vi "Send to Database.vi"(7 "Setting Database In":refnum<class "Setting Database.lvclass">, 8 "error in":errorcluster, 11 "Archivist in":refnum<class "Archivist.lvclass">) -> (0 "error out":errorcluster, 3 "Archivist out":refnum<class "Archivist.lvclass">, 5 "Setting Database Out":refnum<class "Setting Database.lvclass">)   [LabVIEW 2019, in "Archivist.lvclass"]
uses:
  Archivist.lvclass
  Settings/Setting Database/Setting Database.lvclass
  Settings/Setting Database/Typedefs/PrivateEvents--Setting Database.Refresh.ctl
  Archivist.lvclass/Archivist.ctl
  Settings/Dot Settings/Dot Settings.lvclass
  C:/Users/Albro/Documents/GitHub/AFM-Lithography/lvsrc/Classes/Settings/ObjectSettings/ObjectSettings.lvclass
  Settings/Funnel Settings/Funnel Settings.lvclass
  Settings/Rectangle Settings/Rectangle Settings.lvclass
  Settings/Path Settings/Path Settings.lvclass
panel:
  out "Numeric 5":i32
  out "Numeric 4":i32
  out "Numeric 3":i32
  out "Numeric 2":i32
  out "Numeric":i32
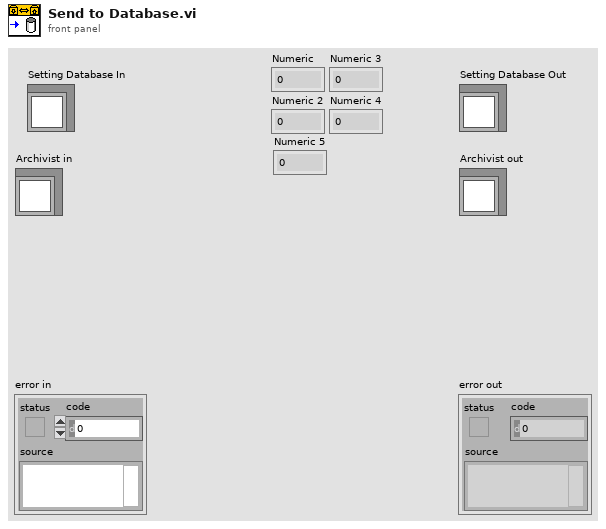
[diagram p1: front panel]
types:
  T1 = typedef "Setting Database.lvclass/PrivateEvents--Setting Database.Refresh.ctl" = cluster{"Paths":string[], "Rectangles":string[], "Funnels":string[], "Dots":string[]}
  T2 = typedef "Setting Database.lvclass/PublicEvents--Setting Database.PathsUpdated.ctl" = refnum<class "Path Settings.lvclass">[]
  T3 = typedef "Setting Database.lvclass/PublicEvents--Setting Database.RectanglesUpdated.ctl" = refnum<class "Rectangle Settings.lvclass">[]
  T4 = typedef "Setting Database.lvclass/PublicEvents--Setting Database.FunnelsUpdated.ctl" = refnum<class "Funnel Settings.lvclass">[]
  T5 = typedef "Setting Database.lvclass/PublicEvents--Setting Database.DotsUpdated.ctl" = refnum<class "Dot Settings.lvclass">[]
  T6 = typedef "Setting Database.lvclass/PublicEvents--Cluster.ctl" = cluster{"NewActivePath":refnum<user-event>, "PathsUpdated":refnum<user-event>, "RectanglesUpdated":refnum<user-event>, "NewActiveRectangle":refnum<user-event>, "NewActiveFunnel":refnum<user-event>, "FunnelsUpdated":refnum<user-event>, "NewActiveDot":refnum<user-event>, "DotsUpdated":refnum<user-event>}
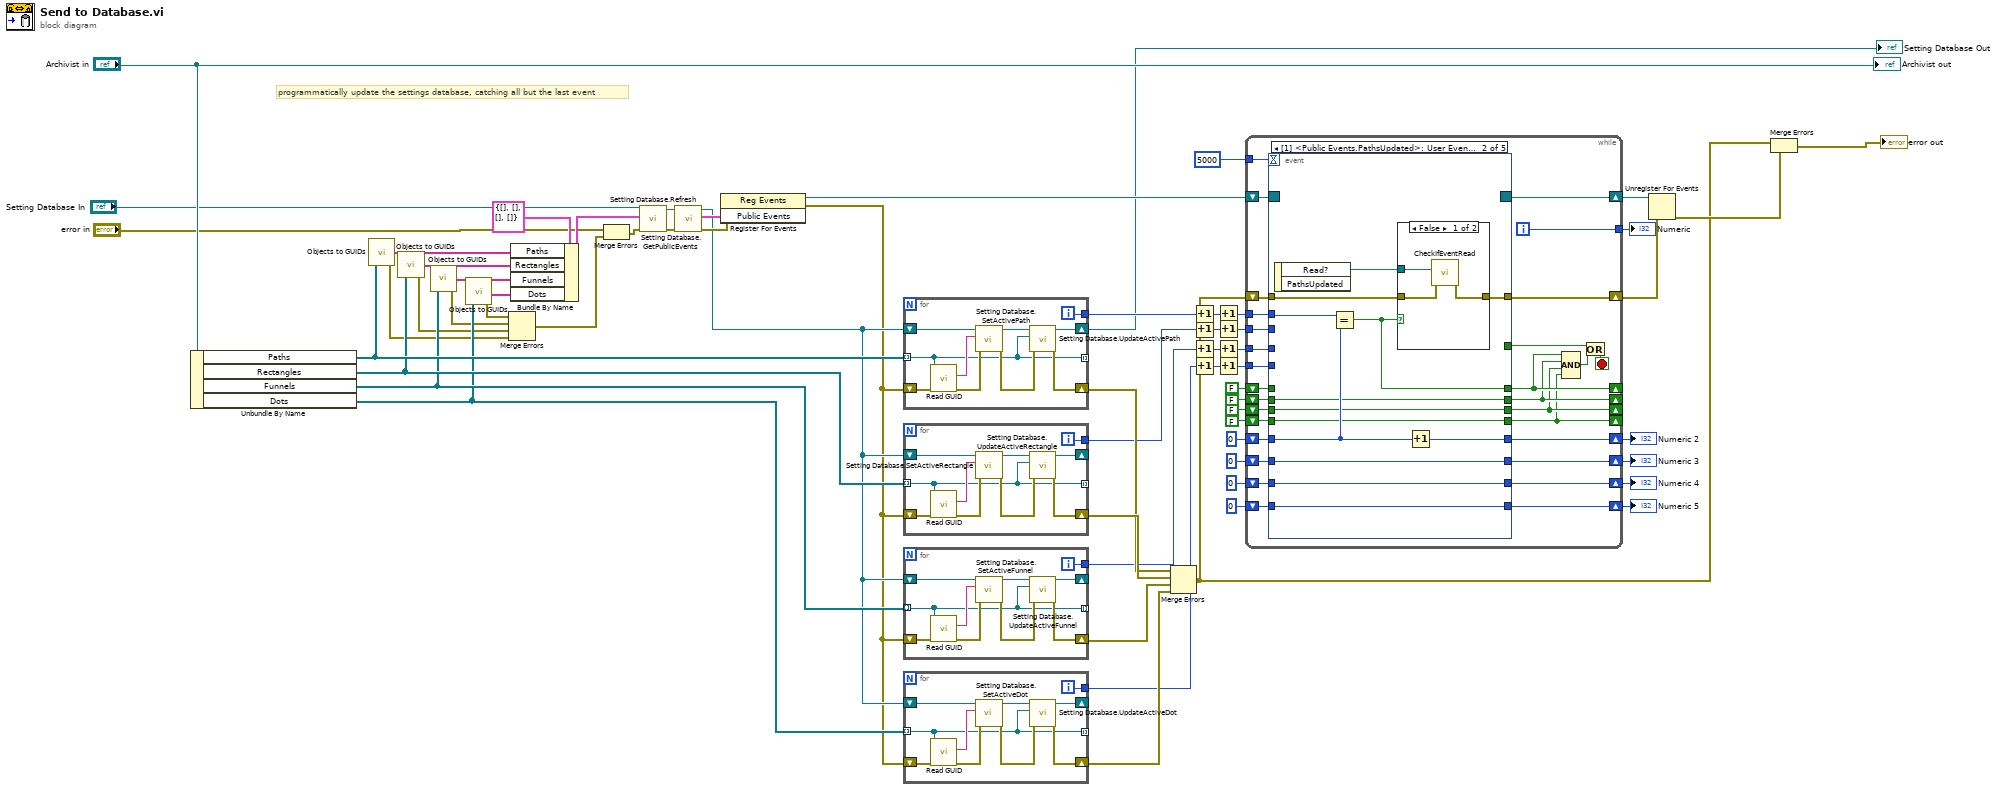
[diagram p0: block diagram]
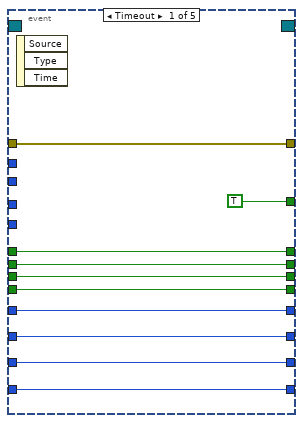
[diagram p2: hidden frame]
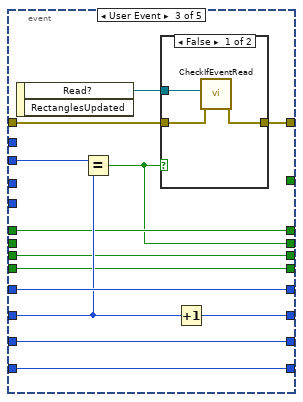
[diagram p4: hidden frame]
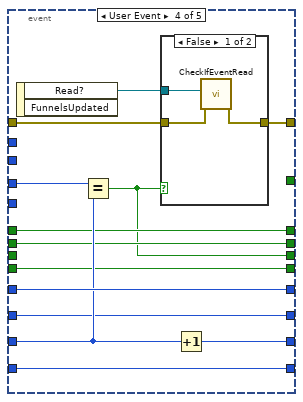
[diagram p6: hidden frame]
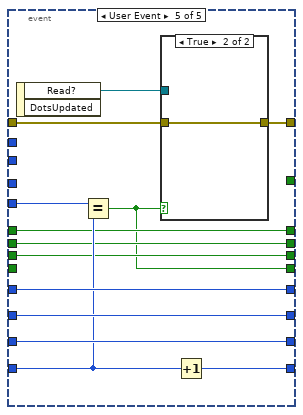
[diagram p8: hidden frame]
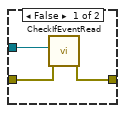
[diagram p9: hidden frame]
diagram:
  # "programmatically update the settings database, catching all but the last event"
  n1 = Unbundle By Name("Archivist in") -> ("Paths"=w51:T2, "Rectangles"=w43:T3, "Funnels"=w42:T4, "Dots"=w41:T5)
  n2 = call "Objects to GUIDs.vi"("Objects"=w51) -> ("error out"=w27:errorcluster, "GUIDs"=w59:string[])  [unwired: 3 in]
  n3 = call "Objects to GUIDs.vi"("Objects"=w43) -> ("error out"=w28:errorcluster, "GUIDs"=w50:string[])  [unwired: 3 in]
  n4 = call "Objects to GUIDs.vi"("Objects"=w42) -> ("error out"=w29:errorcluster, "GUIDs"=w49:string[])  [unwired: 3 in]
  n5 = call "Objects to GUIDs.vi"("Objects"=w41) -> ("error out"=w30:errorcluster, "GUIDs"=w48:string[])  [unwired: 3 in]
  n6 = Merge Errors(w30, w29, w28, w27) -> (w25:errorcluster)
  n7 = Bundle By Name(cluster=T1 {"Paths"=[], "Rectangles"=[], "Funnels"=[], "Dots"=[]} ("Initialize"), "Paths"=w59, "Rectangles"=w50, "Funnels"=w49, "Dots"=w48) -> (w58:T1)
  n8 = Merge Errors("error in", w25) -> (w26:errorcluster)
  n9 = call "Setting Database.Refresh.vi"("error in (no error)"=w26, "Initialize"=w58, "Setting Database"="Setting Database In") -> ("error out"=w45:errorcluster, "Setting Database out"=w46:refnum<class "Setting Database.lvclass">)  [unwired: 7 in]
  n10 = call "Setting Database.GetPublicEvents.vi"("error in (no error)"=w45, "Setting Database"=w46) -> ("error out"=w44:errorcluster, "Public Events"=w47:T6, "Setting Database out"=w40:refnum<class "Setting Database.lvclass">)  [unwired: 7 in]
  n11 = register-events(error in=w44, w47) -> (reference out=w62:refnum<event-registration>, error out=w39:errorcluster)  [unwired: 1 in]
  n12 = for {
    shift-right: [w71] -> w31
    shift-left: w40 -> [w70]
    shift-right: [w66] -> w52
    shift-left: w39 -> [w72]
    tunnel: w51 -> [w64] mode=indexing
    tunnel: [w64] -> _ mode=indexing
    tunnel: [w63] -> w57
    i -> [w63]
    n13 = call-dynamic "Read GUID.vi"("error in (no error)"=w72, "ObjectSettings in"=w64) -> ("error out"=w67:errorcluster, "GUID"=w65:string)  [unwired: 7 in, 1 out]
    n14 = call "Setting Database.SetActivePath.vi"("error in (no error)"=w67, "SetActivePath"=w65, "Setting Database"=w70) -> ("error out"=w68:errorcluster, "Setting Database out"=w69:refnum<class "Setting Database.lvclass">)  [unwired: 7 in]
    n15 = call "Setting Database.UpdateActivePath.vi"("error in (no error)"=w68, "UpdateCurrentPath"=w64, "Setting Database"=w69) -> ("error out"=w66:errorcluster, "Setting Database out"=w71:refnum<class "Setting Database.lvclass">)  [unwired: 7 in]
  }
  "Setting Database Out" <- w31
  n16 = for {
    shift-right: [w81] -> _
    shift-left: w40 -> [w80]
    shift-right: [w76] -> w55
    shift-left: w39 -> [w82]
    tunnel: w43 -> [w74] mode=indexing
    tunnel: [w74] -> _ mode=indexing
    tunnel: [w73] -> w38
    i -> [w73]
    n17 = call-dynamic "Read GUID.vi"("error in (no error)"=w82, "ObjectSettings in"=w74) -> ("error out"=w77:errorcluster, "GUID"=w75:string)  [unwired: 7 in, 1 out]
    n18 = call "Setting Database.SetActiveRectangle.vi"("error in (no error)"=w77, "SetActiveRectangle"=w75, "Setting Database"=w80) -> ("error out"=w78:errorcluster, "Setting Database out"=w79:refnum<class "Setting Database.lvclass">)  [unwired: 7 in]
    n19 = call "Setting Database.UpdateActiveRectangle.vi"("error in (no error)"=w78, "UpdateActiveRectangle"=w74, "Setting Database"=w79) -> ("error out"=w76:errorcluster, "Setting Database out"=w81:refnum<class "Setting Database.lvclass">)  [unwired: 7 in]
  }
  n20 = for {
    shift-right: [w91] -> _
    shift-left: w40 -> [w90]
    shift-right: [w86] -> w54
    shift-left: w39 -> [w92]
    tunnel: w42 -> [w84] mode=indexing
    tunnel: [w84] -> _ mode=indexing
    tunnel: [w83] -> w34
    i -> [w83]
    n21 = call-dynamic "Read GUID.vi"("error in (no error)"=w92, "ObjectSettings in"=w84) -> ("error out"=w87:errorcluster, "GUID"=w85:string)  [unwired: 7 in, 1 out]
    n22 = call "Setting Database.SetActiveFunnel.vi"("error in (no error)"=w87, "SetActiveFunnel"=w85, "Setting Database"=w90) -> ("error out"=w88:errorcluster, "Setting Database out"=w89:refnum<class "Setting Database.lvclass">)  [unwired: 7 in]
    n23 = call "Setting Database.UpdateActiveFunnel.vi"("error in (no error)"=w88, "UpdateActiveFunnel"=w84, "Setting Database"=w89) -> ("error out"=w86:errorcluster, "Setting Database out"=w91:refnum<class "Setting Database.lvclass">)  [unwired: 7 in]
  }
  n24 = for {
    shift-right: [w101] -> _
    shift-left: w40 -> [w100]
    shift-right: [w96] -> w53
    shift-left: w39 -> [w102]
    tunnel: w41 -> [w94] mode=indexing
    tunnel: [w94] -> _ mode=indexing
    tunnel: [w93] -> w33
    i -> [w93]
    n25 = call-dynamic "Read GUID.vi"("error in (no error)"=w102, "ObjectSettings in"=w94) -> ("error out"=w97:errorcluster, "GUID"=w95:string)  [unwired: 7 in, 1 out]
    n26 = call "Setting Database.SetActiveDot.vi"("error in (no error)"=w97, "SetActiveDot"=w95, "Setting Database"=w100) -> ("error out"=w98:errorcluster, "Setting Database out"=w99:refnum<class "Setting Database.lvclass">)  [unwired: 7 in]
    n27 = call "Setting Database.UpdateActiveDot.vi"("error in (no error)"=w98, "UpdateActiveDot"=w94, "Setting Database"=w99) -> ("error out"=w96:errorcluster, "Setting Database out"=w101:refnum<class "Setting Database.lvclass">)  [unwired: 7 in]
  }
  n28 = Merge Errors(w52, w55, w54, w53) -> (w6:errorcluster)
  n29 = Increment(x=w57) -> (x+1=w11:i32)
  n30 = Increment(x=w38) -> (x+1=w10:i32)
  n31 = Increment(x=w34) -> (x+1=w9:i32)
  n32 = Increment(x=w33) -> (x+1=w8:i32)
  n33 = Increment(x=w11) -> (x+1=w1:i32)
  n34 = Increment(x=w10) -> (x+1=w2:i32)
  n35 = Increment(x=w9) -> (x+1=w3:i32)
  n36 = Increment(x=w8) -> (x+1=w4:i32)
  n37 = while {
    shift-right: [w130] -> w24
    shift-left: w62 -> [w131]
    shift-right: [w128] -> w20
    shift-left: 0 -> [w129]
    tunnel: w1 -> [w127]
    shift-right: [w125] -> w22
    shift-left: w6 -> [w126]
    tunnel: w2 -> [w124]
    shift-right: [w123] -> w19
    shift-left: 0 -> [w122]
    shift-right: [w120] -> w18
    shift-left: 0 -> [w121]
    shift-right: [w119] -> w17
    shift-left: 0 -> [w118]
    tunnel: w3 -> [w117]
    tunnel: w4 -> [w116]
    tunnel: [w115] -> w21
    shift-right: [w110] -> _
    shift-left: FALSE -> [w114]
    shift-right: [w109] -> _
    shift-left: FALSE -> [w113]
    shift-right: [w108] -> _
    shift-left: FALSE -> [w112]
    shift-right: [w107] -> _
    shift-left: FALSE -> [w111]
    tunnel: 5000 -> [w106]
    i -> [w115]
    stop <- w104 stop-if-true
    n38 = event shown="[1] <Public Events.PathsUpdated>: User Event" {
      selector: w131 -> [_ _ _ _ _]
      dyn-events: [_ _ _ _ _] -> w130
      timeout: w106 -> [_ _ _ _ _]
      tunnel: w129 -> [w141 w149 w168 w185 w202]
      tunnel: [w141 w152 w168 w185 w202] -> w128
      tunnel: w127 -> [_ w153 _ _ _]
      tunnel: w126 -> [w137 w151 w170 w187 w204]
      tunnel: [w137 w150 w169 w186 w203] -> w125
      tunnel: w124 -> [_ _ w165 _ _]
      tunnel: w122 -> [w140 w148 w164 w181 w200]
      tunnel: [w140 w148 w163 w181 w200] -> w123
      tunnel: w121 -> [w139 w147 w167 w182 w201]
      tunnel: [w139 w147 w167 w180 w201] -> w120
      tunnel: w118 -> [w138 w146 w166 w184 w199]
      tunnel: [w138 w146 w166 w184 w198] -> w119
      tunnel: w117 -> [_ _ _ w183 _]
      tunnel: w116 -> [_ _ _ _ w197]
      tunnel: [w136 w145 w162 w179 w196] -> w110
      tunnel: w114 -> [w136 _ w162 w179 w196]
      tunnel: [w135 w144 w159 w178 w195] -> w109
      tunnel: w113 -> [w135 w144 _ w178 w195]
      tunnel: [w134 w143 w161 w176 w194] -> w108
      tunnel: w112 -> [w134 w143 w161 _ w194]
      tunnel: [w133 w142 w160 w177 w193] -> w107
      tunnel: w111 -> [w133 w142 w160 w177 _]
      tunnel: [TRUE _ _ _ _] -> w103
      event Timeout {
        n39 = event-data() -> ()  [unwired: 1 in, 3 out]
      }
      event User Event {
        n40 = event-data() -> ("Read?"=w154:refnum<notifier>)  [unwired: 1 in, 1 out]
        n41 = Equal?(x=w153, y=w149) -> (x = y?=w145:bool)
        n42 = case shown="False" w145 {
          tunnel: w154 -> [w157 _]
          tunnel: w151 -> [w156 w158]
          tunnel: [w155 w158] -> w150
          frame False {
            n43 = call "CheckIfEventRead.vi"("error in (no error)"=w156, "Read?"=w157) -> ("error out"=w155:errorcluster)  [unwired: 8 in, 1 out]
          }
          frame True {
          }
        }
        n44 = Increment(x=w149) -> (x+1=w152:i32)
      }
      event User Event {
        n45 = event-data() -> ("Read?"=w171:refnum<notifier>)  [unwired: 1 in, 1 out]
        n46 = Equal?(x=w165, y=w164) -> (x = y?=w159:bool)
        n47 = case shown="False" w159 {
          tunnel: w171 -> [w174 _]
          tunnel: w170 -> [w173 w175]
          tunnel: [w172 w175] -> w169
          frame False {
            n48 = call "CheckIfEventRead.vi"("error in (no error)"=w173, "Read?"=w174) -> ("error out"=w172:errorcluster)  [unwired: 8 in, 1 out]
          }
          frame True {
          }
        }
        n49 = Increment(x=w164) -> (x+1=w163:i32)
      }
      event User Event {
        n50 = event-data() -> ("Read?"=w188:refnum<notifier>)  [unwired: 1 in, 1 out]
        n51 = Equal?(x=w183, y=w182) -> (x = y?=w176:bool)
        n52 = case shown="False" w176 {
          tunnel: w188 -> [w191 _]
          tunnel: w187 -> [w190 w192]
          tunnel: [w189 w192] -> w186
          frame False {
            n53 = call "CheckIfEventRead.vi"("error in (no error)"=w190, "Read?"=w191) -> ("error out"=w189:errorcluster)  [unwired: 8 in, 1 out]
          }
          frame True {
          }
        }
        n54 = Increment(x=w182) -> (x+1=w180:i32)
      }
      event User Event {
        n55 = event-data() -> ("Read?"=w205:refnum<notifier>)  [unwired: 1 in, 1 out]
        n56 = Equal?(x=w197, y=w199) -> (x = y?=w193:bool)
        n57 = case shown="True" w193 {
          tunnel: w205 -> [w208 _]
          tunnel: w204 -> [w207 w209]
          tunnel: [w206 w209] -> w203
          frame False {
            n58 = call "CheckIfEventRead.vi"("error in (no error)"=w207, "Read?"=w208) -> ("error out"=w206:errorcluster)  [unwired: 8 in, 1 out]
          }
          frame True {
          }
        }
        n59 = Increment(x=w199) -> (x+1=w198:i32)
      }
    }
    n60 = Compound Arithmetic op=AND(w110, w109, w108, w107) -> (w105:bool)
    n61 = Or(x=w103, y=w105) -> (x .or. y?=w104:bool)
  }
  "Numeric" <- w21
  "Numeric 2" <- w20
  "Numeric 3" <- w19
  "Numeric 4" <- w18
  "Numeric 5" <- w17
  n62 = Unregister For Events(event registration refnum=w24, error in=w22) -> (error out=w23:errorcluster)
  n63 = Merge Errors(w6, w23) -> (→"error out":errorcluster)
  "Archivist out" <- "Archivist in"
